vi "Read Property.vi"(6 "Initialized in":bool, 8 "error in (no error)":errorcluster, 9 "Programming Mode In":T2[](array[typedef]), 10 "References":refnum<vi>[](array[refnum]), 11 "Refnum in":refnum<k20>) -> (0 "error out":errorcluster, 1 "Programming Mode Out":T2[](array[typedef]), 2 "Slot":i32, 3 "Refnum out":refnum<k20>, 4 "Initialized Out":bool)   [LabVIEW 2017, in "Scan Engine Custom Device.lvlib"]
doc: "Get values available (taking into account Model), Read current property value for populated slots, set respective Control."
uses:
  Scan Engine Custom Device.lvlib
  Modules.lvlibp/RSI Module/Module Models.ctl
  Type Defs/Slot - Slot Programming Mode.ctl
  Type Defs/Slot Programming Mode.ctl
  <resource>/objmgr/motionsysapi.rc
  Modules.lvlibp/RSI Module/RSI Module.lvclass
panel:
  in  "Module Name":string
  in  "Slot":T1
  in  "Module":T3
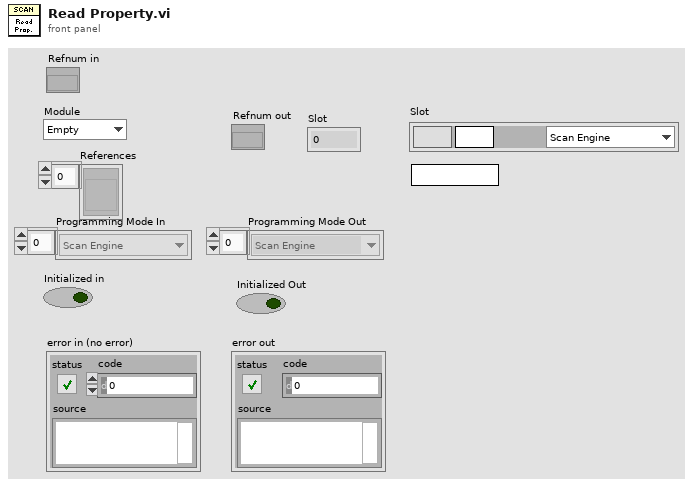
[diagram p1: front panel]
types:
  T1 = typedef "Scan Engine Custom Device.lvlib/Slot - Slot Programming Mode.ctl" = cluster{"Slot":string, "Module Name":string, "Slot Programming Mode":enum16{"Scan Engine", "LabVIEW FPGA", "NI-DAQmx", "Don't Modify"}}
  T2 = typedef "Scan Engine Custom Device.lvlib/Slot Programming Mode.ctl" = enum16{"Scan Engine", "LabVIEW FPGA", "NI-DAQmx", "Don't Modify"}
  T3 = typedef "Modules.lvlibp/RSI Module.lvclass/Module Models.ctl" = enum16{"Empty", "NI 9201", "NI 9203", "NI 9205", "NI 9206", "NI 9207", "NI 9208", "NI 9211", "NI 9212", "NI 9213", "NI 9214", "NI 9215", "NI 9217", "NI 9219", "NI 9220", "NI 9221", "NI 9222", "NI 9223", "NI 9225", "NI 9227", "NI 9229", "NI 9233", "NI 9234", "NI 9235", "NI 9236", "NI 9237", "NI 9239", "NI 9242", "NI 9244", "NI 9263", "NI 9264", "NI 9265", "NI 9266", "NI 9269", "NI 9375", "NI 9401", "NI 9402", "NI 9403", "NI 9411", "NI 9421", "NI 9422", "NI 9423", "NI 9425", "NI 9426", "NI 9435", "NI 9437", "NI 9472", "NI 9474", "NI 9475", "NI 9476", "NI 9477", "NI 9478", "NI 9481", "NI 9482", "NI 9485"}
  T4 = enum8{"Enabled", "Disabled", "Disabled and Grayed Out"}
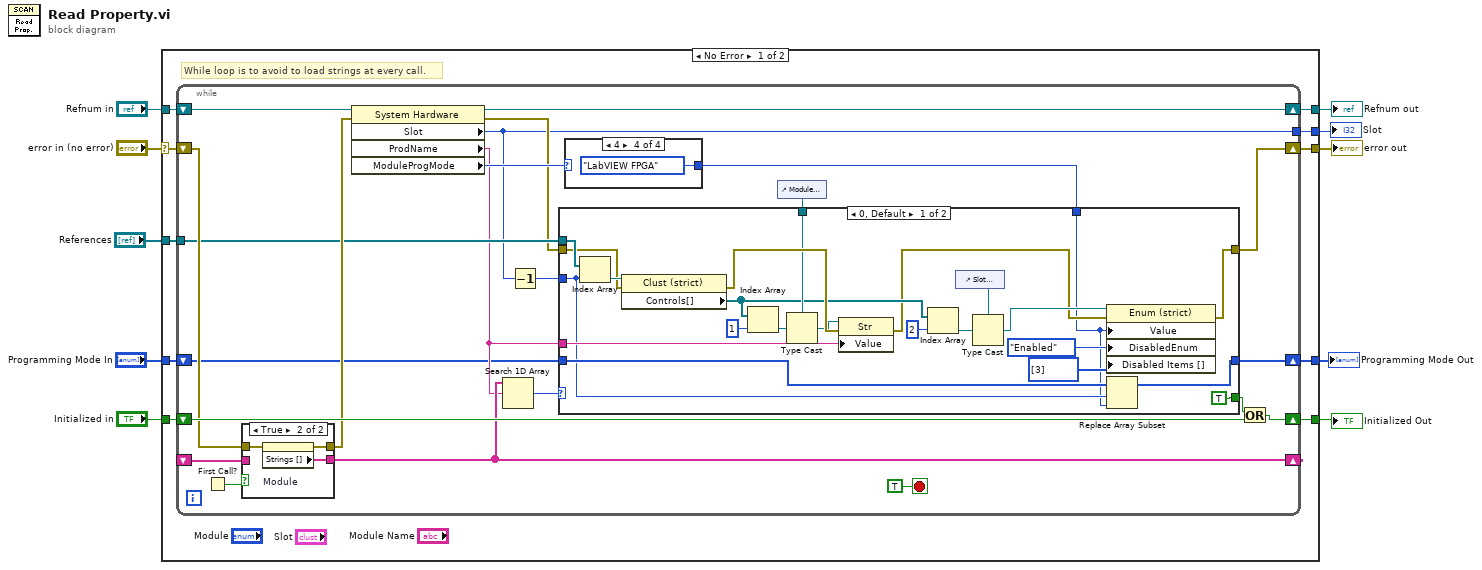
[diagram p0: block diagram]
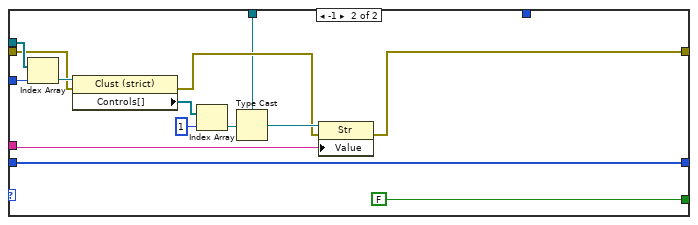
[diagram p2: hidden frame]
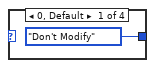
[diagram p4: hidden frame]
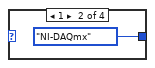
[diagram p5: hidden frame]
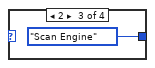
[diagram p6: hidden frame]
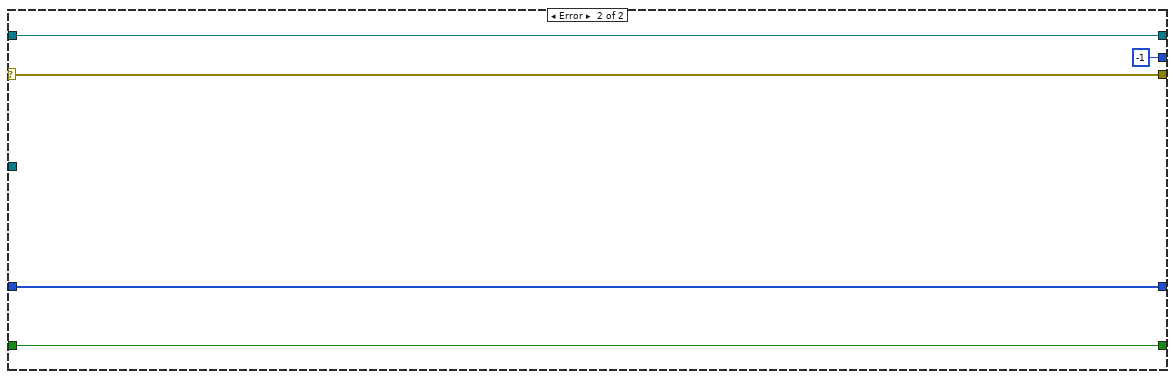
[diagram p7: hidden frame]
diagram:
  n1 = case shown="No Error" "error in (no error)" {
    selector: "error in (no error)" -> [w15 w93]
    tunnel: [w20 w92] -> w10
    tunnel: "Initialized in" -> [w19 w92]
    tunnel: [w18 w93] -> w8
    tunnel: [w17 w94] -> w7
    tunnel: "Refnum in" -> [w16 w94]
    tunnel: "References" -> [w14 _]
    tunnel: "Programming Mode In" -> [w13 w91]
    tunnel: [w12 w91] -> w2
    tunnel: [w11 -1 ("Slot")] -> w1
    frame No Error {
      # "While loop is to avoid to load strings at every call."
      n2 = while {
        shift-right: [w43] -> w20
        shift-left: w19 -> [w42]
        shift-right: [w40] -> w17
        shift-left: w16 -> [w39]
        shift-right: [w32] -> w18
        shift-left: w15 -> [w34]
        shift-right: [w33] -> _
        shift-left: _ -> [w35]
        tunnel: w14 -> [w30]
        shift-right: [w25] -> w12
        shift-left: w13 -> [w26]
        tunnel: [w21] -> w11
        stop <- TRUE stop-if-true
        n3 = First Call?() -> (First Call?: T/F=w37:bool)
        n4 = case shown="True" w37 {
          tunnel: [w82 w85] -> w36
          tunnel: [w81 w84] -> w33
          tunnel: w35 -> [w81 _]
          tunnel: w34 -> [w82 w83]
          frame False {
          }
          frame True {
            n5 = property on="Module" class="Enum (strict)"(error in=w83) -> (error out=w85:errorcluster, "Strings []"=w84:string[])  [unwired: 1 in, 1 out]
          }
        }
        n6 = property class="System Hardware"(reference=w39, error in=w36) -> (reference out=w40:refnum<k20>, error out=w28:errorcluster, "Slot"=w21:i32, "ProdName"=w27:string, "ModuleProgMode"=w29:u32)
        n7 = Search 1D Array(1D array=w33, element=w27) -> (index of element=w31:i32)  [unwired: 1 in]
        n8 = Decrement(x=w21) -> (x-1=w22:i32)
        n9 = case shown="4" w29 {
          tunnel: [Slot_Programming_Mode."Don't Modify" ("Value") Slot_Programming_Mode."NI-DAQmx" ("Value") Slot_Programming_Mode."Scan Engine" ("Value") Slot_Programming_Mode."LabVIEW FPGA" ("Value")] -> w23
          frame 0, Default {
          }
          frame 1 {
          }
          frame 2 {
          }
          frame 4 {
          }
        }
        n10 = control-ref of="Module Name"() -> (w24:refnum<vi>)
        n11 = case shown="0, Default" w31 {
          tunnel: [TRUE FALSE] -> w41
          tunnel: w28 -> [w59 w75]
          tunnel: [w49 w69] -> w32
          tunnel: w30 -> [w60 w78]
          tunnel: w22 -> [w46 w77]
          tunnel: w27 -> [w57 w68]
          tunnel: w26 -> [w47 w79]
          tunnel: [w44 w79] -> w25
          tunnel: w24 -> [w58 w67]
          tunnel: w23 -> [w45 _]
          frame 0, Default {
            n12 = Index Array(array=w60, index=w46) -> (element=w62:refnum<vi>)
            n13 = property class="Clust (strict)"(reference=w62, error in=w59) -> (error out=w65:errorcluster, "Controls[]"=w56:refnum<vi>[])  [unwired: 1 out]
            n14 = Index Array(array=w56, index=1) -> (element=w63:refnum<vi>)
            n15 = Type Cast(type=w58, x=w63) -> (*(type *) &x=w64:refnum<vi>)
            n16 = property class="Str"(reference=w64, error in=w65, "Value"=w57) -> (error out=w50:errorcluster)  [unwired: 1 out]
            n17 = Index Array(array=w56, index=2) -> (element=w54:refnum<vi>)
            n18 = control-ref of="Slot Programming Mode"() -> (w53:refnum<vi>)
            n19 = Type Cast(type=w53, x=w54) -> (*(type *) &x=w51:refnum<vi>)
            n20 = property class="Enum (strict)"(reference=w51, error in=w50, "Value"=w45, "DisabledEnum"=T4."Enabled" ("Disabled"), "Disabled Items []"=i32[] [3]) -> (error out=w49:errorcluster)  [unwired: 1 out]
            n21 = Replace Array Subset(array=w47, new element=w45, index=w46) -> (w44:T2[])
          }
          frame -1 {
            n22 = Index Array(array=w78, index=w77) -> (element=w76:refnum<vi>)
            n23 = property class="Clust (strict)"(reference=w76, error in=w75) -> (error out=w70:errorcluster, "Controls[]"=w74:refnum<vi>[])  [unwired: 1 out]
            n24 = Index Array(array=w74, index=1) -> (element=w72:refnum<vi>)
            n25 = Type Cast(type=w67, x=w72) -> (*(type *) &x=w71:refnum<vi>)
            n26 = property class="Str"(reference=w71, error in=w70, "Value"=w68) -> (error out=w69:errorcluster)  [unwired: 1 out]
          }
        }
        n27 = Or(x=w41, y=w42) -> (x .or. y?=w43:bool)
      }
    }
    frame Error {
    }
  }
  "Initialized Out" <- w10
  "error out" <- w8
  "Refnum out" <- w7
  "Programming Mode Out" <- w2
  "Slot" <- w1
